vi "Pre Launch Init.vi"(11 "通讯 in":refnum<class "通讯.lvclass"> caption="操作者输入") -> (0 "error out":errorcluster caption="错误输出", 3 "通讯 out":refnum<class "通讯.lvclass"> caption="操作者输出")   [LabVIEW 2015, in "通讯.lvlib" / "通讯.lvclass"]
doc: "(<B>文件名</B>: Actor Framework.lvlib:Actor.lvclass:Pre Launch Init.vi)\n\n定义启动嵌套操作者方法被调用之后、操作者核心方法开始运行之前的操作。\n\n默认情况下，该方法不执行任何操作。子孙类重写该方法定义具体的操作。"
uses:
  <vilib>/ActorFramework/Actor/Actor.lvclass
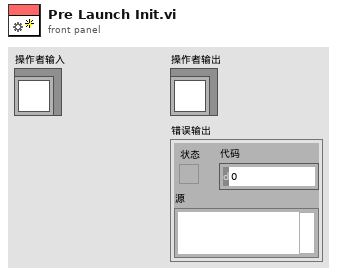
[diagram p1: front panel]
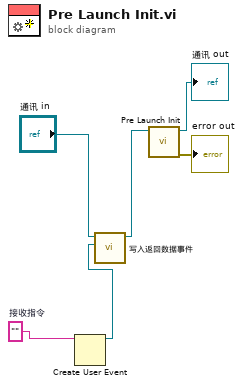
[diagram p0: block diagram]
diagram:
  w3 = ""  # 接收指令
  n1 = Create User Event(user event datatype=w3) -> (user event=w2:refnum<user-event>)  [unwired: 1 in, 1 out]
  n2 = call-dynamic "写入返回数据事件.vi"("返回数据事件"=w2, "通讯输入"="通讯 in") -> ("通讯输出"=w1:refnum<class "通讯.lvclass">)  [unwired: 8 in, 1 out]
  n3 = call-parent "Pre Launch Init.vi"("Actor in"=w1) -> ("error out"=→"error out":errorcluster, "Actor out"=→"通讯 out":refnum<class "通讯.lvclass">)  [unwired: 9 in]
